vi "Configure Trace Type.vi"(7 "Trace Format (0: ASCii)":i32(ring) items=["ASCii", "Real"], 8 "error in (no error)":errorcluster, 9 "Trace (1: Trace 1)":i32(ring)=1 items=["Trace 1"=1, "Trace 2"=2, "Trace 3"=3, "Trace 4"=4], 10 "Trace Type (0: Write)":i32(ring) items=["Write", "Maximum hold", "Minimum hold", "View", "Blank"], 11 "VISA resource name":refnum<visa-resource-name>) -> (0 "error out":errorcluster, 3 "VISA resource name out":refnum<visa-resource-name>)   [LabVIEW 2022 SP3, in "Agilent N934X Series.lvlib"]
doc: "Configures the type of trace to acquire."
uses:
  <instrlib>/Agilent N934X Series/Agilent N934X Series.lvlib
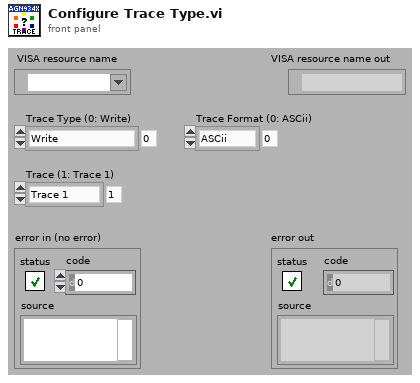
[diagram p1: front panel]
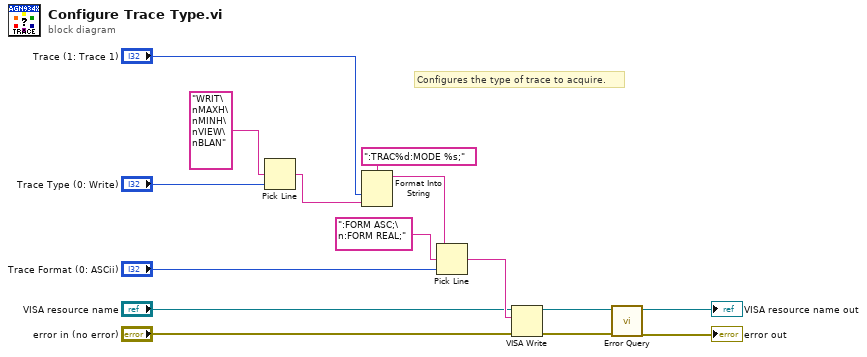
[diagram p0: block diagram]
diagram:
  # "Configures the type of trace to acquire."
  n1 = Pick Line(multi-line string="WRIT\nMAXH\nMINH\nVIEW\nBLAN", line index="Trace Type (0: Write)") -> (output string=w11:string)  [unwired: 1 in]
  n2 = Format Into String(format string=":TRAC%d:MODE %s;", "Trace (1: Trace 1)", w11) -> (resulting string=w8:string)  [unwired: 2 in, 1 out]
  n3 = Pick Line(string ("")=w8, multi-line string=":FORM ASC;\n:FORM REAL;", line index="Trace Format (0: ASCii)") -> (output string=w7:string)
  n4 = VISA Write(VISA resource name="VISA resource name", write buffer=w7, error in (no error)="error in (no error)") -> (VISA resource name out=w4:refnum<visa-resource-name>, error out=w3:errorcluster)  [unwired: 1 out]
  n5 = call <instrlib>:"Error Query.vi"("error in (no error)"=w3, "VISA resource name"=w4) -> ("error out"=→"error out":errorcluster, "VISA resource name out"=→"VISA resource name out":refnum<visa-resource-name>)  [unwired: 6 in, 2 out]
